vi "Large integer U8 array - max # of shifts.vi"(3 "LI-U8 B":T1, 5 "LI-U8 A":T1) -> (0 "LI-U8 shifted B":T1, 1 "Max # shifts (U8)":u8)   [LabVIEW 2013]
doc: "Determines the maxinum # of LEFT (higher value) base 256 shifts that can be applied to B and still have A greater than B"
uses:
  User Access Type defs/Large number - U8 array.ctl
panel:
  # "index 0 = LSD"
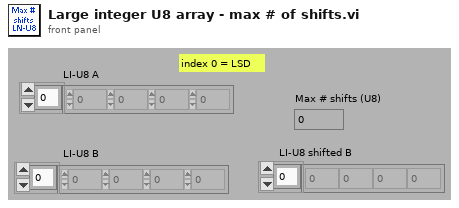
[diagram p1: front panel]
types:
  T1 = typedef "Large number - U8 array.ctl" = u8[]
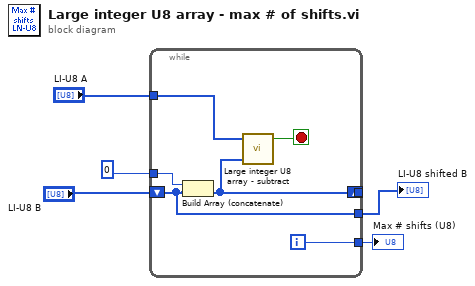
[diagram p0: block diagram]
diagram:
  n1 = while {
    shift-right: [w7] -> _
    shift-left: "LI-U8 B" -> [w6]
    tunnel: [w10] -> w5
    tunnel: [w7] -> _
    tunnel: u8 0 ("Numeric") -> [w9]
    tunnel: "LI-U8 A" -> [w8]
    tunnel: [w6] -> w1
    i -> [w10]
    stop <- w11 stop-if-true
    n2 = Build Array (concatenate)(w9, w6) -> (w7:T1)
    n3 = call "Large integer U8 array - subtract.vi"("Large number - U8 B"=w7, "Large number - U8 A"=w8) -> ("Overflow?"=w11:bool)  [unwired: 3 out]
  }
  "Max # shifts (U8)" <- w5
  "LI-U8 shifted B" <- w1
